vi "Get Time.vi"(8 "error in (no error)":errorcluster, 11 "VISA resource name":refnum<visa-resource-name>) -> (0 "error out":errorcluster, 2 "output":i32, 3 "VISA resource name out":refnum<visa-resource-name>)   [LabVIEW 2025, in "Detector SCPI.lvlib"]
doc: "Gets timing of last BURST read\nReturns time to take reading in usec"
uses:
  Detector SCPI.lvlib
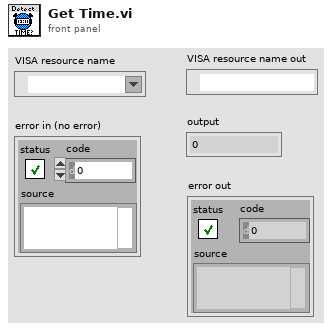
[diagram p1: front panel]
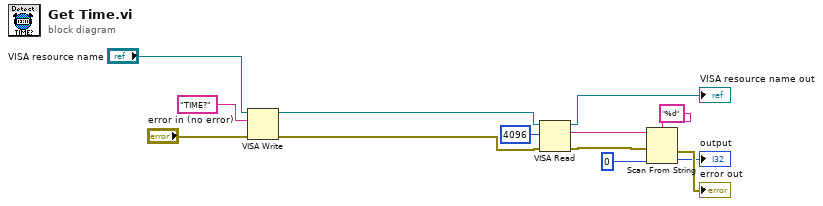
[diagram p0: block diagram]
diagram:
  n1 = VISA Write(VISA resource name="VISA resource name", write buffer="TIME?" ("command"), error in (no error)="error in (no error)") -> (VISA resource name out=w1:refnum<visa-resource-name>, error out=w11:errorcluster)  [unwired: 1 out]
  n2 = VISA Read(VISA resource name=w1, byte count=u32 4096, error in (no error)=w11) -> (VISA resource name out=→"VISA resource name out":refnum<visa-resource-name>, read buffer=w7:string, error out=w5:errorcluster)  [unwired: 1 out]
  n3 = Scan From String(format string="%d", input string=w7, error in=w5, default 1=0 ("default value 1")) -> (error out=→"error out":errorcluster, output 1=→"output":i32)  [unwired: 1 in, 2 out]
